vi "LIA Post Build.vi"() -> ()   [LabVIEW 2023]
uses:
  <userlib>/Levylab/Build Support/PostBuildSupport/PostBuildSupport.lvclass
  <userlib>/_OpenG.lib/file/file.llb/openg_file.lvlib
panel:
  in  "Package Version":string="4.59.10"
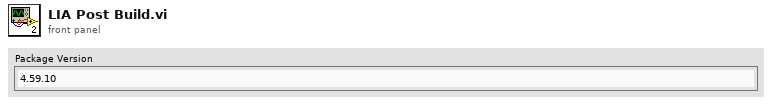
[diagram p1: front panel]
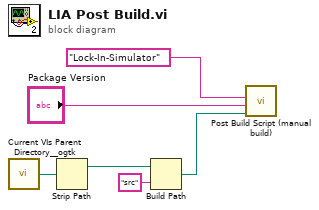
[diagram p0: block diagram]
diagram:
  n1 = call <userlib>:"Current VIs Parent Directory__ogtk.vi"() -> ("Parent Directory (+ Relative)"=w6:path)  [unwired: 5 in]
  n2 = Strip Path(path=w6) -> (stripped path=w5:path)  [unwired: 1 out]
  n3 = Build Path(base path=w5, name or relative path="src") -> (appended path=w1:path)
  n4 = call <userlib>:"Post Build Script (manual build).vi"("Package Source Folder"=w1, "Package Version"="Package Version", "Product Name"="Lock-In-Simulator") -> ()  [unwired: 8 in, 1 out]
